vi "DBLoop.vi"() -> ()   [LabVIEW 2014, in "DBLoop.lvlib"]
uses:
  DBLoop.lvlib
  <vilib>/addons/database/NI_Database_API.lvlib
  <vilib>/addons/database/_DB Variant To Data/Database Variant To Data.xnode
  APIs/Message Queue/WINFAS 2 Message Queue.lvlib
  <vilib>/addons/database/Connection.llb/DB Tools Open Connec (String).vi
  <vilib>/addons/database/Connection.llb/Conn ObjectReference.ctl
  APIs/Data Queue/Acquisition Data 1 Sample Cluster.ctl
  APIs/Data Queue/WINFAS 2 Data Queue.lvlib
  APIs/Data Queue/Control Data Cluster.ctl
  APIs/Data Queue/Async Acquisition Data Cluster.ctl
  APIs/Data Queue/All Data Queues Cluster.ctl
  APIs/Message Queue/Message Cluster.ctl
panel:
  out "error out":errorcluster
  in  "error in (no error)":errorcluster
  in  "DB":refnum<queue>
  in  "CORE":refnum<queue>
  in  "ACQ Data Queue":T1
  in  "Server":string
  in  "Password":string
  in  "User ID":string
  out "Display Core Pressure & Temperature":string[][](table)
  out "Display max pressure value":dbl format="%#.6g"
  out "Display min pressure value":dbl format="%#.6g"
  out "Display max temperature value":dbl format="%#.6g"
  out "Display min temperature value":dbl format="%#.6g"
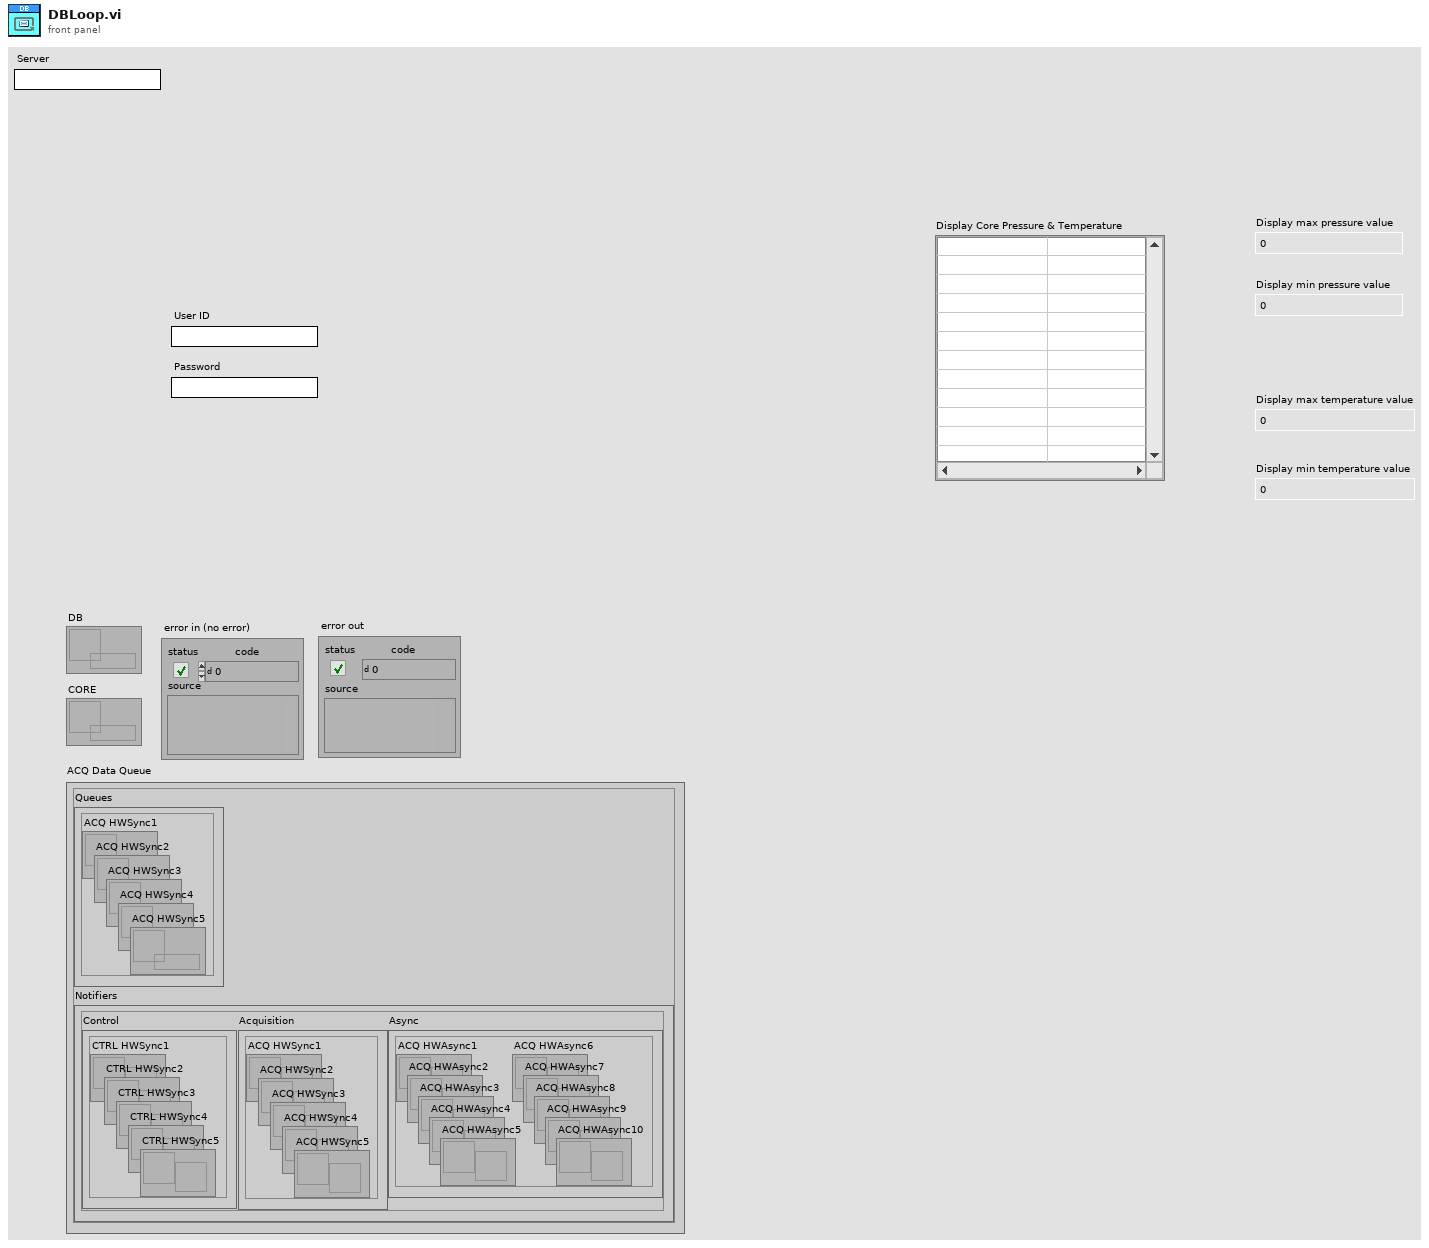
[diagram p1: front panel]
types:
  T1 = typedef "WINFAS 2 Data Queue.lvlib/All Data Queues Cluster.ctl" = cluster{"Queues":cluster{"ACQ HWSync1":refnum<queue>, "ACQ HWSync2":refnum<queue>, "ACQ HWSync3":refnum<queue>, "ACQ HWSync4":refnum<queue>, "ACQ HWSync5":refnum<queue>}, "Notifiers":cluster{"Control":cluster{"CTRL HWSync1":refnum<notifier>, "CTRL HWSync2":refnum<notifier>, "CTRL HWSync3":refnum<notifier>, "CTRL HWSync4":refnum<notifier>, "CTRL HWSync5":refnum<notifier>}, "Acquisition":cluster{"ACQ HWSync1":refnum<notifier>, "ACQ HWSync2":refnum<notifier>, "ACQ HWSync3":refnum<notifier>, "ACQ HWSync4":refnum<notifier>, "ACQ HWSync5":refnum<notifier>}, "Async":cluster{"ACQ HWAsync1":refnum<notifier>, "ACQ HWAsync2":refnum<notifier>, "ACQ HWAsync3":refnum<notifier>, "ACQ HWAsync4":refnum<notifier>, "ACQ HWAsync5":refnum<notifier>, "ACQ HWAsync6":refnum<notifier>, "ACQ HWAsync7":refnum<notifier>, "ACQ HWAsync8":refnum<notifier>, "ACQ HWAsync9":refnum<notifier>, "ACQ HWAsync10":refnum<notifier>}}}
  T2 = typedef "NI_Database_API.lvlib/Conn ObjectReference.ctl" = refnum<k1>
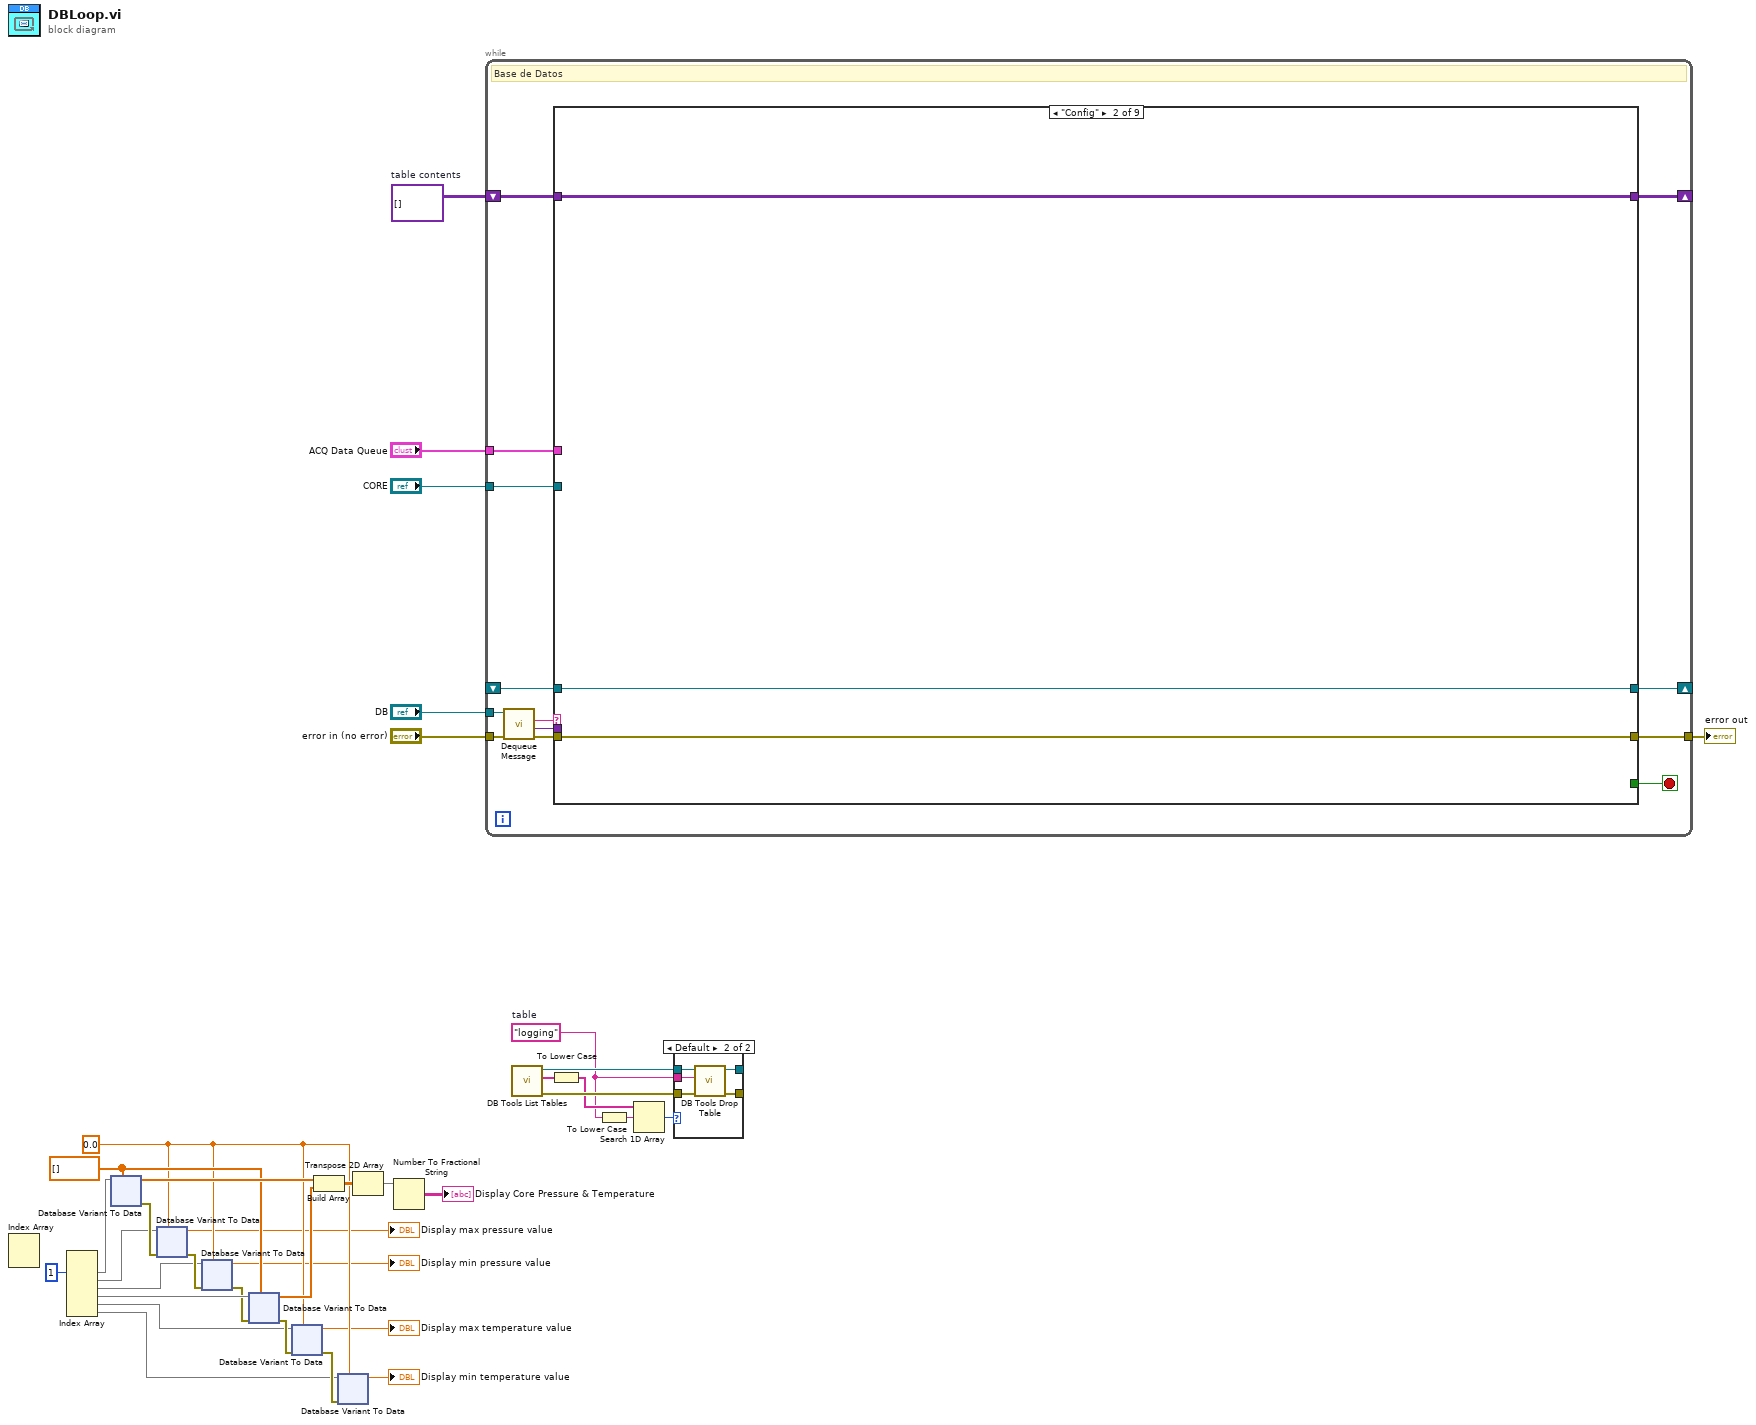
[diagram p0: block diagram]
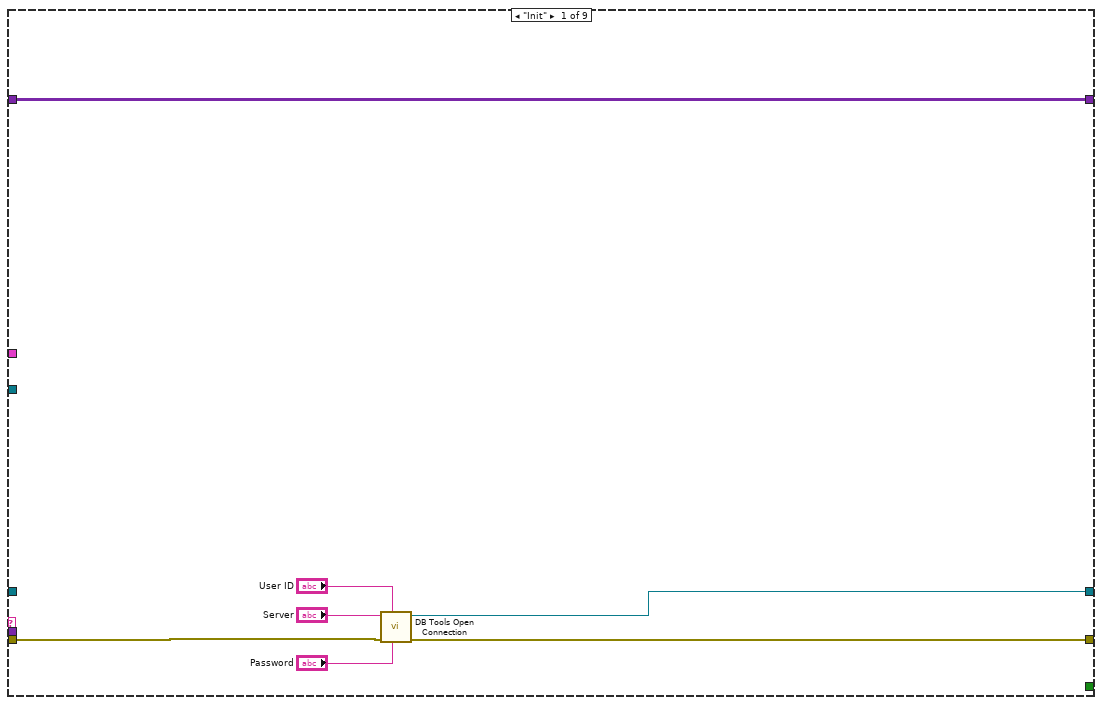
[diagram p2: hidden frame]
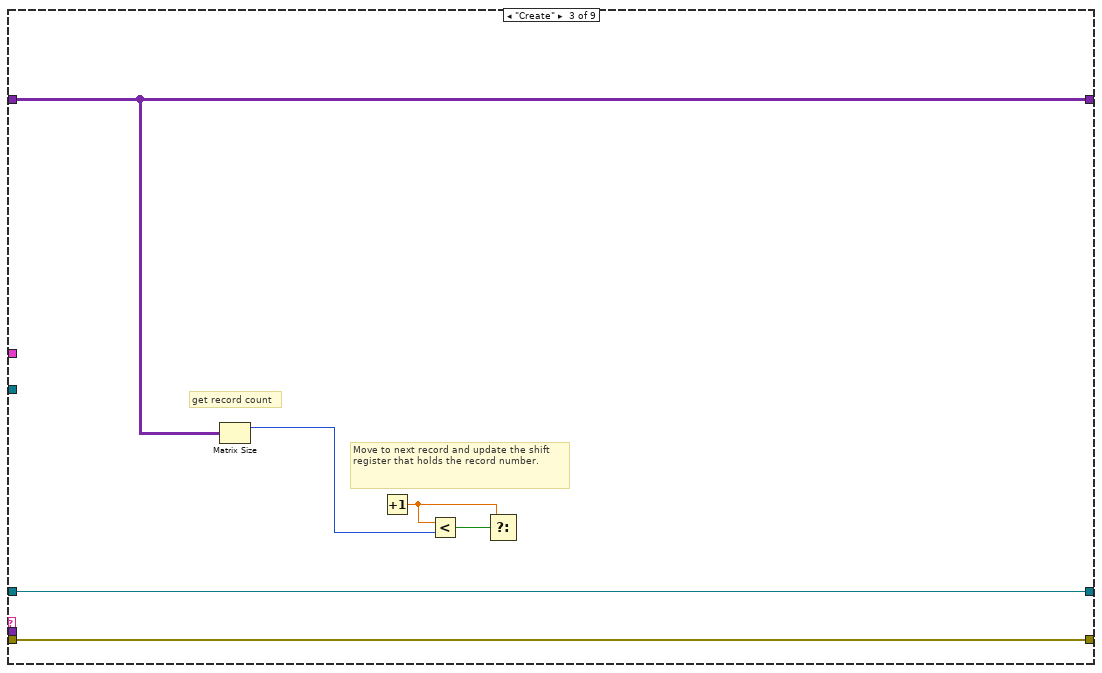
[diagram p3: hidden frame]
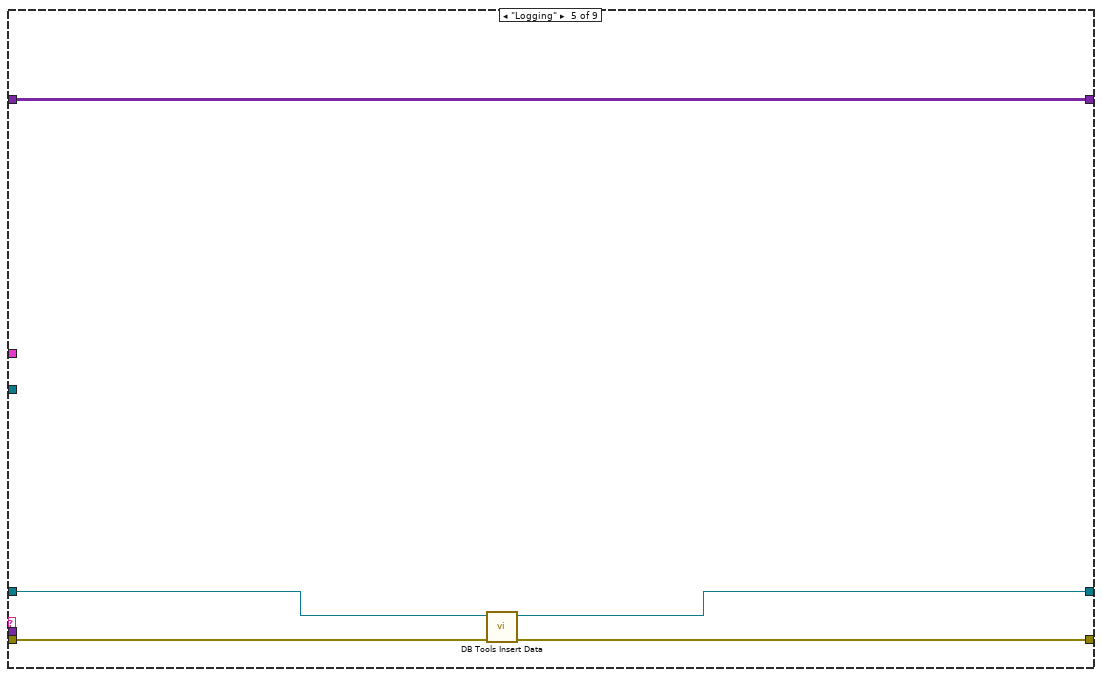
[diagram p5: hidden frame]
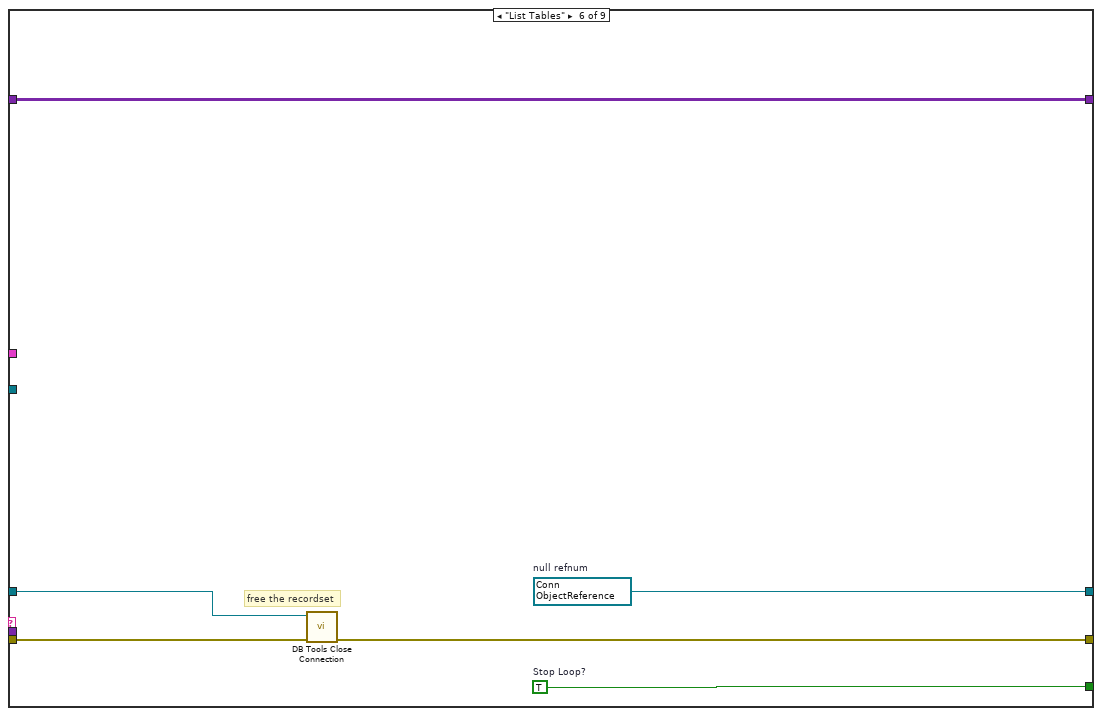
[diagram p6: hidden frame]
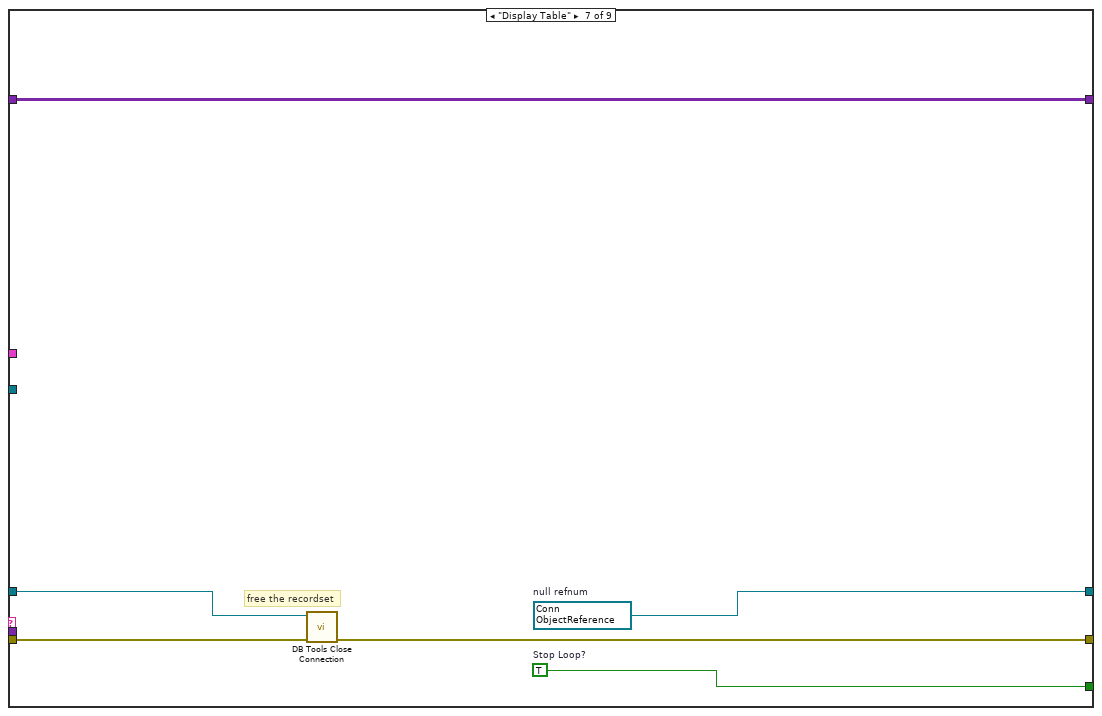
[diagram p7: hidden frame]
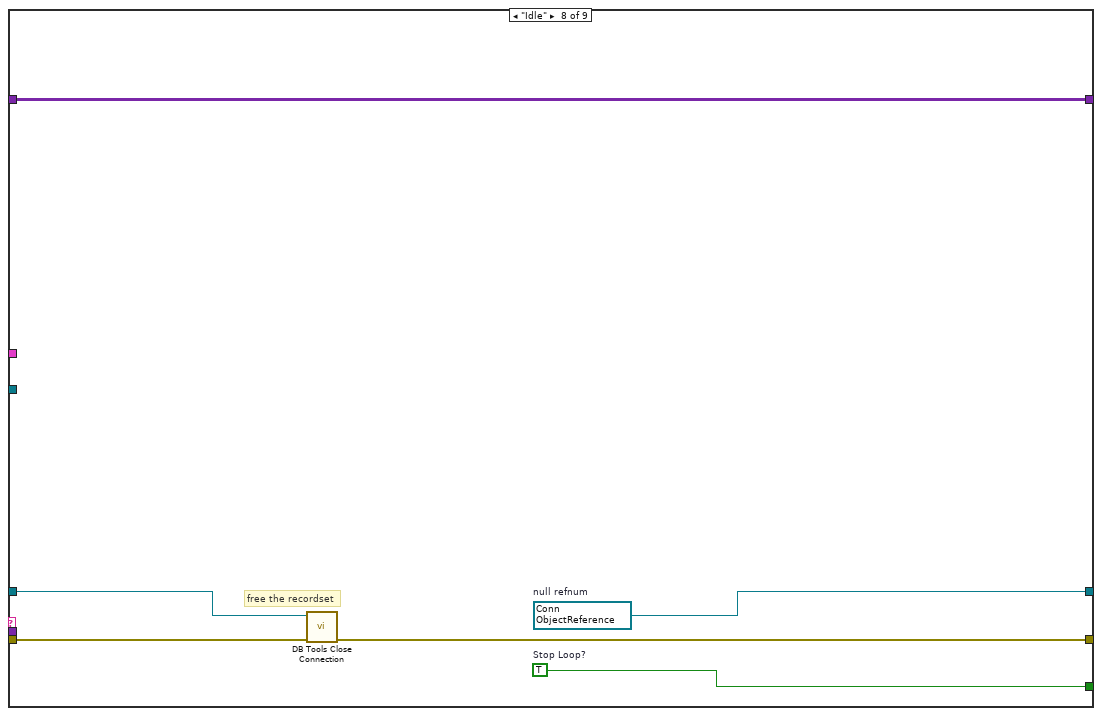
[diagram p8: hidden frame]
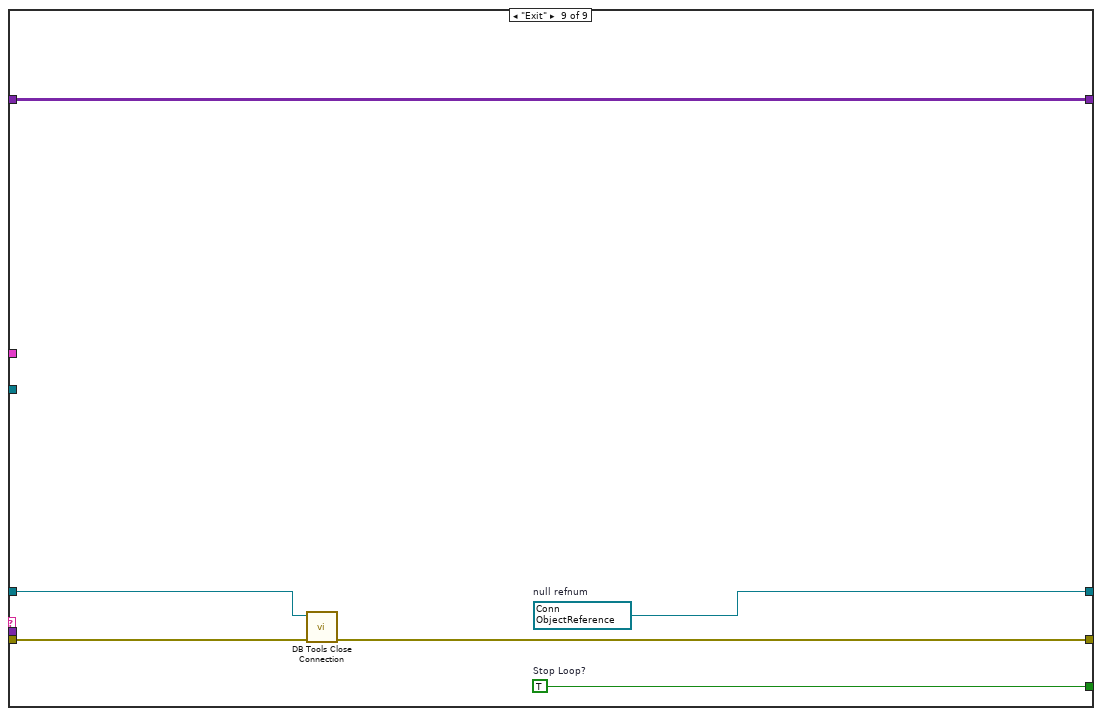
[diagram p9: hidden frame]
diagram:
  w21 = 0.0
  w23 = dbl[] [] ("Array Constant")
  w29 = variant[][] []  # table contents
  w30 = "logging"  # table
  n1 = Index Array() -> ()  [unwired: 3 in, 1 out]
  n2 = Index Array(index #1=1) -> (element #1=w12, element #2=w11, element #3=w10, element #4=w9, element #5=w8, element #6=w7)  [unwired: 6 in]
  n3 = xnode "Database Variant To Data"("database variant"=w12, "type"=w23) -> ("data"=w28:dbl[], "error out"=w13:errorcluster)  [unwired: 1 in]
  n4 = xnode "Database Variant To Data"("database variant"=w11, "error in (no error)"=w13, "type"=w21) -> ("data"=→"Display max pressure value":dbl, "error out"=w15:errorcluster)
  n5 = xnode "Database Variant To Data"("database variant"=w10, "error in (no error)"=w15, "type"=w21) -> ("data"=→"Display min pressure value":dbl, "error out"=w6:errorcluster)
  n6 = xnode "Database Variant To Data"("database variant"=w9, "error in (no error)"=w6, "type"=w23) -> ("data"=w24:dbl[], "error out"=w14:errorcluster)
  n7 = xnode "Database Variant To Data"("database variant"=w8, "error in (no error)"=w14, "type"=w21) -> ("data"=→"Display max temperature value":dbl, "error out"=w20:errorcluster)
  n8 = Build Array(w28, w24) -> (w25:dbl[][])
  n9 = xnode "Database Variant To Data"("database variant"=w7, "error in (no error)"=w20, "type"=w21) -> ("data"=→"Display min temperature value":dbl)  [unwired: 1 out]
  n10 = Transpose 2D Array(2D array=w25) -> (transposed array=w26:dbl[][])
  n11 = Number To Fractional String(number=w26) -> (F-format string=→"Display Core Pressure & Temperature":string[][])  [unwired: 3 in]
  n12 = while {
    shift-right: [w48] -> _
    shift-left: _ -> [w47]
    shift-right: [w46] -> _
    shift-left: w29 -> [w45]
    tunnel: "DB" -> [w43]
    tunnel: [w49] -> w4
    tunnel: "error in (no error)" -> [w41]
    tunnel: "CORE" -> [w39]
    tunnel: "ACQ Data Queue" -> [w38]
    stop <- w40 stop-if-true
    # "Base de Datos"
    n13 = call "Dequeue Message.vi"("error in (no error)"=w41, "Message Queue"=w43) -> ("error out"=w42:errorcluster, "Message Data"=w37:variant, "Message"=w44:string)  [unwired: 6 in, 1 out]
    n14 = case shown="\"Config\"" w44 {
      tunnel: [_ _ _ _ _ w79 w85 w91 w97] -> w40
      tunnel: w42 -> [w55 w58 w65 w68 w71 w78 w84 w90 w96]
      tunnel: [w54 w58 w65 w68 w70 w77 w83 w89 w95] -> w49
      tunnel: [w53 w59 w64 w67 w72 w75 w81 w87 w94] -> w48
      tunnel: w47 -> [_ w59 w64 w67 w73 w76 w82 w88 w92]
      tunnel: [w56 w57 w61 w66 w69 w74 w80 w86 w93] -> w46
      tunnel: w45 -> [w56 w57 w61 w66 w69 w74 w80 w86 w93]
      tunnel: w39 -> [_ _ _ _ _ _ _ _ _]
      tunnel: w38 -> [_ _ _ _ _ _ _ _ _]
      tunnel: w37 -> [_ _ _ _ _ _ _ _ _]
      frame "Init" {
        n15 = call-poly <vilib>:"DB Tools Open Connection.vi"("password"="Password", "userID"="User ID", "error in (no error)"=w55, "connection information"="Server") -> ("error out"=w54:errorcluster, "connection reference"=w53:T2)  [unwired: 4 in]
      }
      frame "Config" {
      }
      frame "Create" {
        # "get record count"
        # "Move to next record and update the shift register that holds the record number."
        n16 = Matrix Size(0:w61) -> (1:w60:i32)  [unwired: 1 out]
        n17 = Increment() -> (x+1=w63:dbl)  [unwired: 1 in]
        n18 = Less?(x=w63, y=w60) -> (x < y?=w62:bool)
        n19 = Select(t=w63, s=w62) -> ()  [unwired: 1 in, 1 out]
      }
      frame "Delete" {
      }
      frame "Logging" {
        n20 = call <vilib>:"DB Tools Insert Data.vi"("error in (no error)"=w71, "connection reference"=w73) -> ("error out"=w70:errorcluster, "connection reference out"=w72:T2)  [unwired: 8 in]
      }
      frame "List Tables" {
        w75 = T2 refnum items=["Connection"]  # null refnum
        w79 = TRUE  # Stop Loop?
        # "free the recordset"
        n21 = call <vilib>:"DB Tools Close Connection.vi"("error in (no error)"=w78, "connection reference"=w76) -> ("error out"=w77:errorcluster)  [unwired: 5 in]
      }
      frame "Display Table" {
        w81 = T2 refnum items=["Connection"]  # null refnum
        w85 = TRUE  # Stop Loop?
        # "free the recordset"
        n22 = call <vilib>:"DB Tools Close Connection.vi"("error in (no error)"=w84, "connection reference"=w82) -> ("error out"=w83:errorcluster)  [unwired: 5 in]
      }
      frame "Idle" {
        w87 = T2 refnum items=["Connection"]  # null refnum
        w91 = TRUE  # Stop Loop?
        # "free the recordset"
        n23 = call <vilib>:"DB Tools Close Connection.vi"("error in (no error)"=w90, "connection reference"=w88) -> ("error out"=w89:errorcluster)  [unwired: 5 in]
      }
      frame "Exit" {
        w94 = T2 refnum items=["Connection"]  # null refnum
        w97 = TRUE  # Stop Loop?
        n24 = call <vilib>:"DB Tools Close Connection.vi"("error in (no error)"=w96, "connection reference"=w92) -> ("error out"=w95:errorcluster)  [unwired: 5 in]
      }
    }
  }
  "error out" <- w4
  n25 = call <vilib>:"DB Tools List Tables.vi"() -> ("error out"=w35:errorcluster, "tables"=w36:string[], "connection reference out"=w34:T2)  [unwired: 5 in]
  n26 = To Lower Case(string=w36) -> (all lower case string=w33:string[])
  n27 = To Lower Case(string=w30) -> (all lower case string=w32:string)
  n28 = Search 1D Array(1D array=w33, element=w32) -> (index of element=w31:i32)  [unwired: 1 in]
  n29 = case shown="Default" w31 {
    tunnel: w35 -> [w98 w104]
    tunnel: w34 -> [w99 w103]
    tunnel: [w99 w102] -> _
    tunnel: [w98 w101] -> _
    tunnel: w30 -> [_ w100]
    frame -1 {
    }
    frame Default {
      n30 = call <vilib>:"DB Tools Drop Table.vi"("error in (no error)"=w104, "table"=w100, "connection reference"=w103) -> ("error out"=w101:errorcluster, "connection reference out"=w102:T2)  [unwired: 5 in]
    }
  }
